vi "create python session.vi"(8 "error in (no error)":errorcluster) -> (0 "error out":errorcluster, 2 "version num":string, 3 "session out":refnum<k35>)   [LabVIEW 2021, in "Framework_lib.lvlib"]
uses:
  SubVis/QMH/Framework_lib.lvlib
  <vilib>/regexp/Match Regular Expression.xnode
panel:
  out "bitness":string
  out "standard output":string
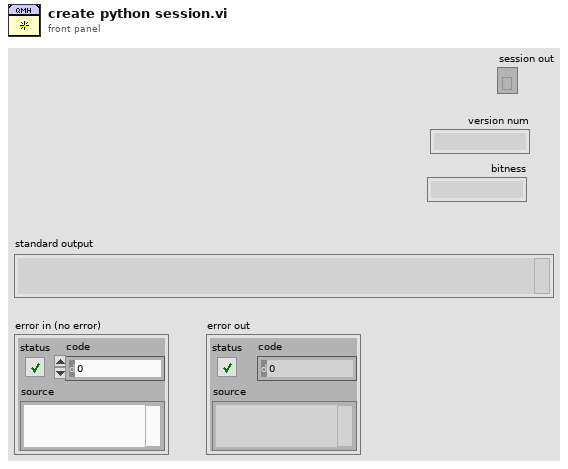
[diagram p1: front panel]
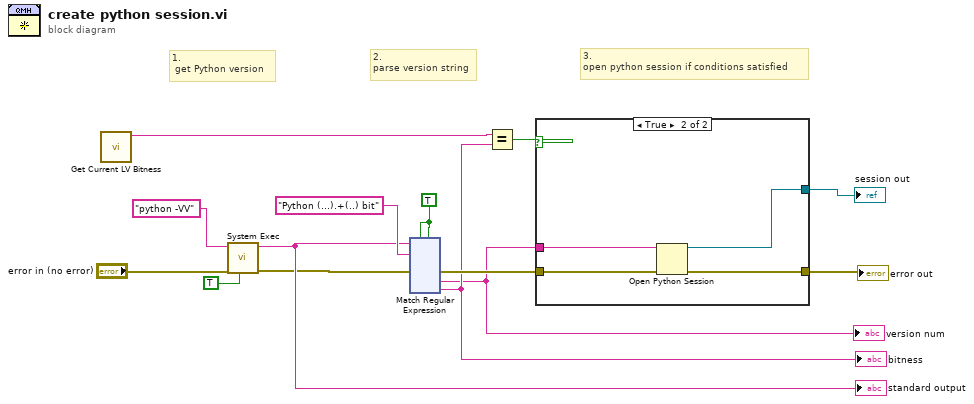
[diagram p0: block diagram]
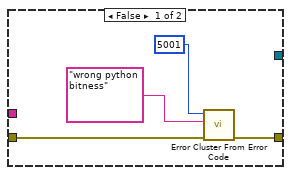
[diagram p2: hidden frame]
diagram:
  w12 = TRUE ("multiline? (F)")
  # "3.\nopen python session if conditions satisfied"
  # "2.\nparse version string"
  # "1.\n get Python version"
  n1 = call <vilib>:"Get Current LV Bitness.vi"() -> ("bitness"=w5:string)  [unwired: 11 in]
  n2 = call <vilib>:"System Exec.vi"("run minimized? (F)"=TRUE, "error in (no error)"="error in (no error)", "command line"="python -VV") -> ("error out"=w10:errorcluster, "standard output"=w11:string)  [unwired: 5 in, 2 out]
  "standard output" <- w11
  n3 = xnode "Match Regular Expression"("input string"=w11, "regular expression"="Python (...).+(..) bit", "error in"=w10, "ignore case? (F)"=w12, "multiline? (F)"=w12) -> ("error out"=w8:errorcluster, "submatch 1"=w2:string, "submatch 2"=w6:string)  [unwired: 1 in, 4 out]
  "version num" <- w2
  "bitness" <- w6
  n4 = Equal?(x=w5, y=w6) -> (x = y?=w4:bool)
  n5 = case shown="True" w4 {
    tunnel: w8 -> [w17 w22]
    tunnel: [w18 w21] -> w7
    tunnel: w2 -> [_ w20]
    tunnel: [_ w19] -> w1
    frame False {
      n6 = call <vilib>:"Error Cluster From Error Code.vi"("error in (no error)"=w17, "error message (\"\")"="wrong python bitness" ("error message (\"\")"), "error code (0)"=5001) -> ("error out"=w18:errorcluster)  [unwired: 6 in]
    }
    frame True {
      n7 = Open Python Session(python version=w20, 3:w22) -> (session out=w19:refnum<k35>, error out=w21:errorcluster)  [unwired: 1 in]
    }
  }
  "error out" <- w7
  "session out" <- w1
